vi "__Select bucket dialog.vi"(1 "Buckets":T1[](array[typedef])) -> (0 "Selected bucket":string)   [LabVIEW 2011]
doc: "This is a dialog, that allows you to select one of the items given in the Buckets string array input."
uses:
  vi.lib/National Instruments/LabVIEW Interface for Amazon S3/Typedefs/AMZ_S3_API_Bucket.ctl
  vi.lib/National Instruments/LabVIEW Interface for Amazon S3/LV Interface for Amazon S3.lvlib
panel:
  in  "Cancel":bool
  in  "OK":bool
  in  "Bucket":string(combo)
  # "Please select the bucket \nyou want to use."
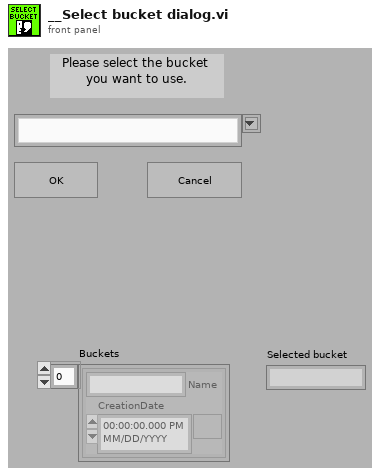
[diagram p1: front panel]
types:
  T1 = typedef "LV Interface for Amazon S3.lvlib/AMZ_S3_API_Bucket.ctl" = cluster{"Name":string, "CreationDate":timestamp}
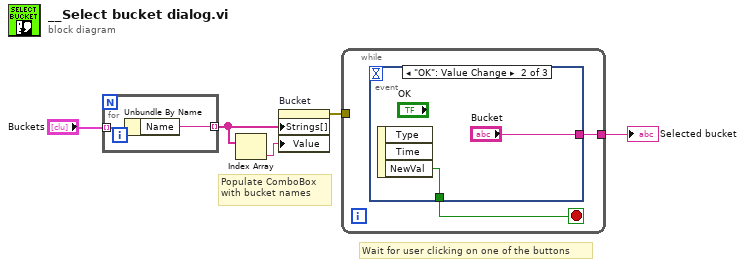
[diagram p0: block diagram]
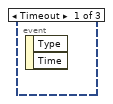
[diagram p2: hidden frame]
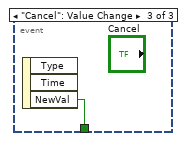
[diagram p3: hidden frame]
diagram:
  # "Wait for user clicking on one of the buttons"
  # "Populate ComboBox\nwith bucket names"
  n1 = for {
    tunnel: "Buckets" -> [w7] mode=indexing
    tunnel: [w6] -> w2 mode=indexing
    n2 = Unbundle By Name(w7) -> ("Name"=w6:string)
  }
  n3 = Index Array(array=w2) -> (element=w1:string)  [unwired: 1 in]
  n4 = property on="Bucket" class="CmbBox"("Strings[]"=w2, "Value"=w1) -> (error out=w4:errorcluster)  [unwired: 2 in, 1 out]
  n5 = while {
    tunnel: w4 -> [_]
    tunnel: [w8] -> w3
    stop <- w9 stop-if-true
    n6 = event shown="[1] \"OK\": Value Change" {
      selector: _ -> [_ _ _]
      dyn-events: _ -> [_ _ _]
      timeout: _ -> [_ _ _]
      tunnel: [_ w11 w12] -> w9
      tunnel: [_ "Bucket" _] -> w8
      event Timeout {
        n7 = event-data() -> ()  [unwired: 1 in, 2 out]
      }
      event "OK": Value Change {
        n8 = event-data() -> ("NewVal"=w11:bool)  [unwired: 1 in, 2 out]
      }
      event "Cancel": Value Change {
        n9 = event-data() -> ("NewVal"=w12:bool)  [unwired: 1 in, 2 out]
      }
    }
  }
  "Selected bucket" <- w3
